vi "QPD1.vi"() -> ()   [LabVIEW 2019]
uses:
  <vilib>/DAQmx/read.llb/DAQmx Read (Analog 2D DBL NChan NSamp).vi
  <vilib>/DAQmx/create/channels.llb/DAQmx Create Channel (AI-Voltage-Basic).vi
  global_VIs/Global_1.vi
  <vilib>/DAQmx/configure/timing.llb/DAQmx Timing (Sample Clock).vi
  <vilib>/DAQmx/miscellaneous.llb/DAQmx Fill In Error Info.vi
panel:
  out "X 4":dynamicdata(graph)
  out "X 3":dynamicdata(graph)
  out "X 2":dynamicdata(graph)
  in  "stop":bool
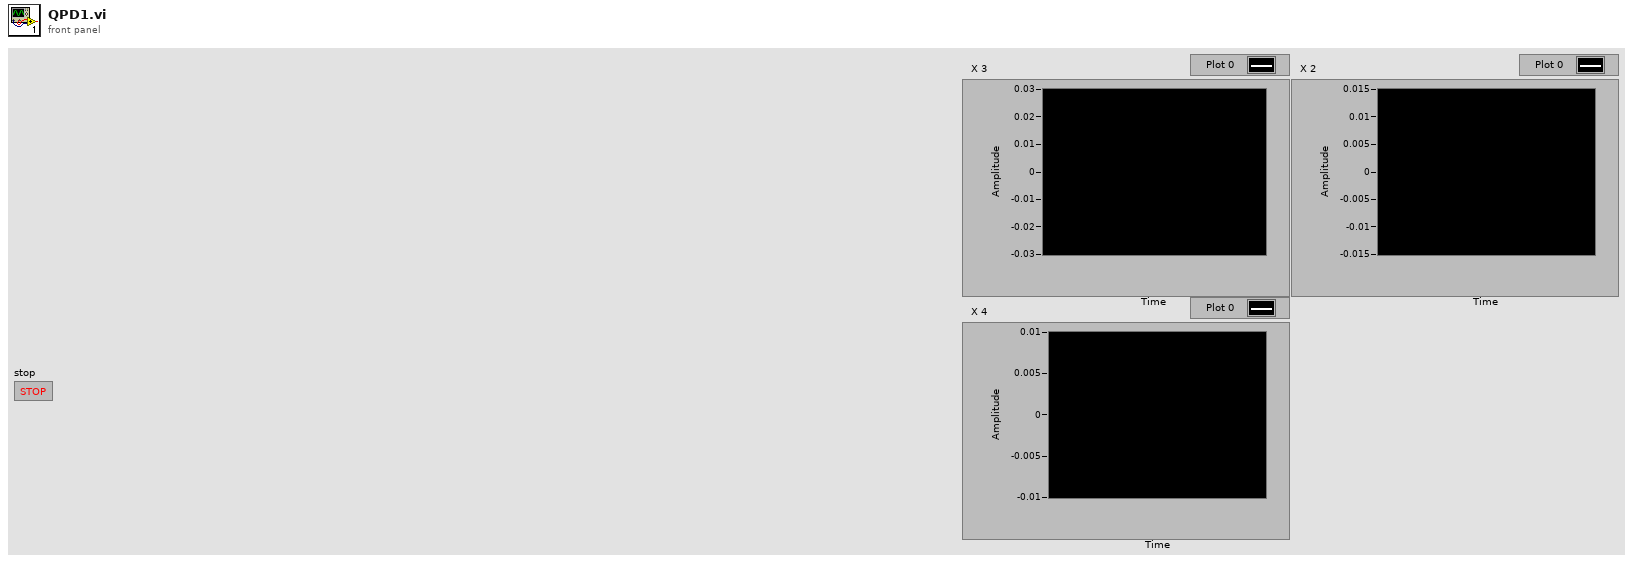
[diagram p1: front panel]
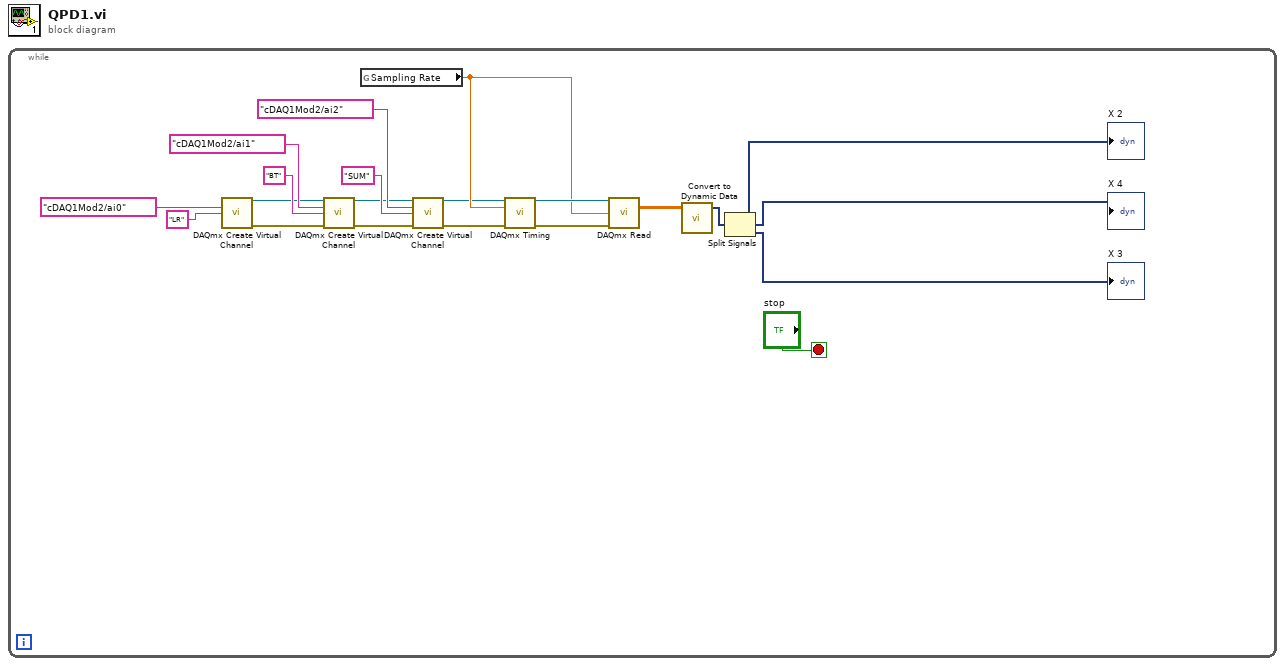
[diagram p0: block diagram]
diagram:
  n1 = while {
    stop <- "stop" stop-if-true
    n2 = call-poly <vilib>:"DAQmx Create Virtual Channel.vi"("physical channels"=tag "cDAQ1Mod2/ai0", "name to assign"="LR") -> ("task out"=w11:refnum<k21>, "error out"=w10:errorcluster)  [unwired: 12 in]
    n3 = call-poly <vilib>:"DAQmx Create Virtual Channel.vi"("task in"=w11, "physical channels"=tag "cDAQ1Mod2/ai1", "name to assign"="BT", "error in"=w10) -> ("task out"=w9:refnum<k21>, "error out"=w8:errorcluster)  [unwired: 10 in]
    n4 = global read "Global_1.vi" "Sampling Rate"() -> (w19:dbl)
    n5 = call-poly <vilib>:"DAQmx Create Virtual Channel.vi"("task in"=w9, "physical channels"=tag "cDAQ1Mod2/ai2", "name to assign"="SUM", "error in"=w8) -> ("task out"=w7:refnum<k21>, "error out"=w6:errorcluster)  [unwired: 10 in]
    n6 = call-poly <vilib>:"DAQmx Timing.vi"("task/channels in"=w7, "rate"=w19, "error in"=w6) -> ("task out"=w20:refnum<k21>, "error out"=w21:errorcluster)  [unwired: 11 in]
    n7 = call-poly <vilib>:"DAQmx Read.vi"("task/channels in"=w20, "number of samples per channel"=w19, "error in"=w21) -> ("data"=w5:dbl[][])  [unwired: 10 in, 2 out]
    n8 = call "Convert to Dynamic Data"("2D Array"=w5) -> ("Dynamic Data Type"=w1:dynamicdata)  [unwired: 3 in]
    n9 = Split Signals(w1) -> (→"X 2":dynamicdata, →"X 4":dynamicdata, →"X 3":dynamicdata)  [unwired: 3 in]
  }
